vi "Read RMS.vi"(8 "error in (no error)":errorcluster, 11 "Roughness Averager in":refnum<class "Roughness Averager.lvclass">) -> (0 "error out":errorcluster, 2 "RMS":dbl, 3 "Roughness Averager out":refnum<class "Roughness Averager.lvclass">)   [LabVIEW 2018, in "Roughness Averager.lvclass"]
uses:
  Roughness Averager.lvclass
  Roughness Averager.lvclass/Roughness Averager.ctl
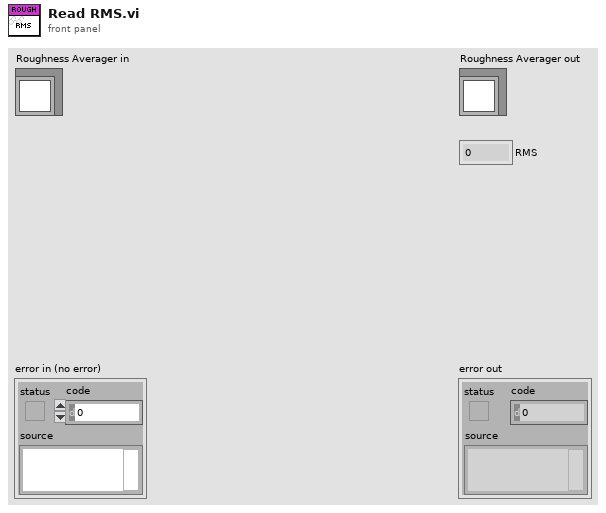
[diagram p1: front panel]
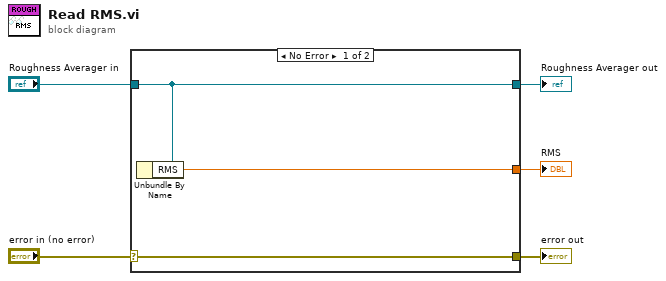
[diagram p0: block diagram]
diagram:
  n1 = case shown="No Error" "error in (no error)" {
    selector: "error in (no error)" -> [w8 w9]
    tunnel: [w8 w9] -> w4
    tunnel: [w7 w10] -> w2
    tunnel: "Roughness Averager in" -> [w7 w10]
    tunnel: [w6 _] -> w1
    frame No Error {
      n2 = Unbundle By Name(w7) -> ("RMS"=w6:dbl)
    }
    frame Error {
    }
  }
  "error out" <- w4
  "Roughness Averager out" <- w2
  "RMS" <- w1
